vi "错误处理.vi"(0 "error in (no error)":errorcluster={"status"=TRUE, "code"=51111, "source"=""}) -> ()   [LabVIEW 2013]
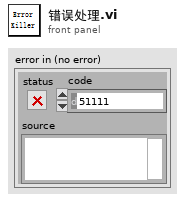
[diagram p1: front panel]
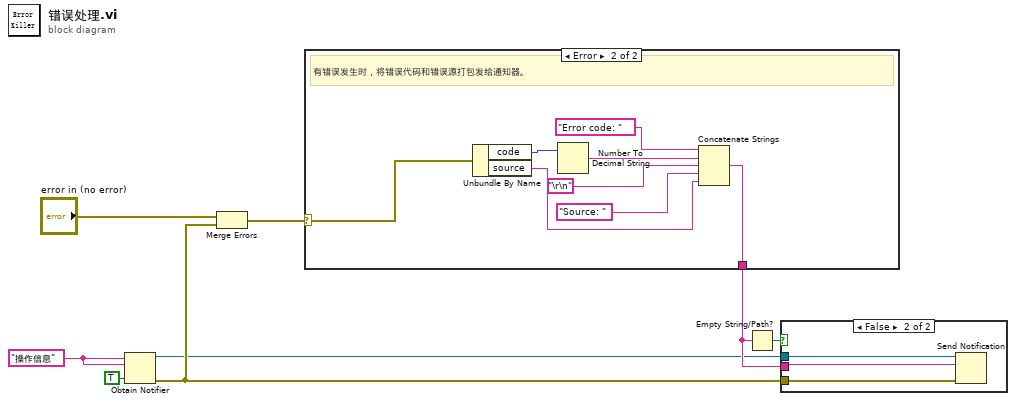
[diagram p0: block diagram]
diagram:
  w8 = "操作信息"
  n1 = Obtain Notifier(name (unnamed)=w8, notification data type=w8, create if not found? (T)=TRUE) -> (notifier out=w1:refnum<notifier>, error out=w2:errorcluster)  [unwired: 1 in, 1 out]
  n2 = Merge Errors("error in (no error)", w2) -> (w5:errorcluster)
  n3 = case shown="Error" w5 {
    selector: w5 -> [_ w10]
    tunnel: [_ w9] -> w3
    frame No Error {
    }
    frame Error {
      # "有错误发生时，将错误代码和错误源打包发给通知器。"
      n4 = Unbundle By Name(w10) -> ("code"=w16:i32, "source"=w12:string)
      n5 = Number To Decimal String(number=w16) -> (decimal integer string=w15:string)  [unwired: 1 in]
      n6 = Concatenate Strings("Error code: ", w15, "\r\n", "Source: ", w12) -> (w9:string)
    }
  }
  n7 = Empty String/Path?(string/path=w3) -> (empty?=w4:bool)
  n8 = case shown="False" w4 {
    tunnel: w1 -> [_ w19]
    tunnel: w3 -> [_ w18]
    tunnel: w2 -> [_ w17]
    frame True {
    }
    frame False {
      n9 = Send Notification(notification=w18, notifier=w19, error in (no error)=w17) -> ()  [unwired: 2 out]
    }
  }
